vi "stm_GetIDfromName_.vi"(9 "Name":string, 11 "MetaData":T1[](array[typedef])) -> (1 "Found":bool, 3 "Meta ID":u16)   [LabVIEW 2010]
doc: "This VI looks up the Meta data index using the Meta data name."
uses:
  stm_MetaDataElement.ctl
  NI STM.lvlib
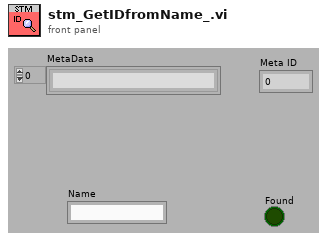
[diagram p1: front panel]
types:
  T1 = typedef "stm_MetaDataElement.ctl" = string
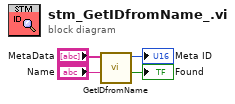
[diagram p0: block diagram]
diagram:
  n1 = call "GetIDfromName.vi"("Name"="Name", "MetaData"="MetaData") -> ("Found"=→"Found":bool, "Meta ID"=→"Meta ID":u16)  [unwired: 8 in]
